vi "Fire Stop Event.vi"(8 "error in":errorcluster) -> (0 "error out":errorcluster)   [LabVIEW 2015, in "Generic Module Library.lvlib" / "Template G_Module.lvlib"]
uses:
  Template G_Module.lvlib
  Private Controls/Event Item.ctl
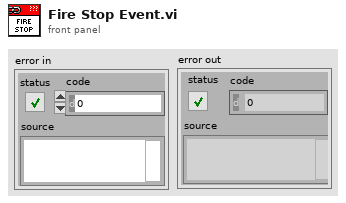
[diagram p1: front panel]
types:
  T1 = typedef "Generic Module Library.lvlib/Template G_Module.lvlib/Event Item.ctl" = cluster{"Event Data":variant}
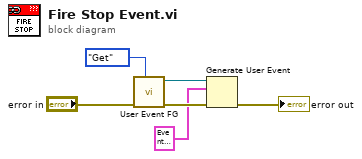
[diagram p0: block diagram]
diagram:
  n1 = call "User Event FG.vi"("User Event Actions"=enum16{"Destroy", "Create", "Get"}."Get", "error in"="error in") -> ("error out"=w5:errorcluster, "Event Item"=w2:refnum<user-event>)  [unwired: 8 in]
  n2 = Generate User Event(user event=w2, event data cluster=T1 {"Event Data"=variant} ("event data"), error in=w5) -> (error out=→"error out":errorcluster)  [unwired: 1 in, 1 out]
